vi "Build Channel Group.vi"(8 "error in":errorcluster, 9 "Selected Group":T1, 11 "Config Grandmaster":T3) -> (0 "error out":errorcluster={"status"=TRUE, "code"=-200220, "source"="Property Node DAQmx Device (arg 2) in ge_BuildGroup.vi <append>\n<B>Device Specified: </B>empty string"}, 1 "Selected Group":T1, 3 "Config Grandmaster":T3, 4 "Canceled?":bool)   [LabVIEW 2018, in "Configuration Grandmaster.lvlib" / "Cfg Grandmaster.lvclass"]
uses:
  Cfg Grandmaster.lvclass
  Custom Ctrls/ge_MeasType.ctl
  Custom Ctrls/Master Cfg/ge_Cfg wChassis.ctl
  Class Chassis Cfg/ChassisCfg.lvclass
  Class Chassis BOM/Chassis BOM.lvclass
  Data Acquisition/Class Chassis Tasks/Chassis Tasks.lvclass
  Common/Controls/Selected Group.ctl
  Common/Controls/TE_Designator.ctl
  Class Chassis BOM/Chassis BOM.lvclass/Chassis BOM.ctl
  <vilib>/Utility/miscctls.llb/LVRowAndColumnTypeDef.ctl
  <vilib>/Utility/miscctls.llb/LVRowAndColumnUnsignedTypeDef.ctl
  Class Chassis BOM/Read Mod Infos.vi
  Class Chassis BOM/Read Chassis Alias.vi
  Class Chan Group/Read GrpName.vi
  Class Chan Group/Read MeasType.vi
  <resource>/objmgr/daqmx.rc
  Measurements/Class Channel/Channel.lvclass
  Class Chan Group/ChanGrp.lvclass
panel:
  in  "Timing Engine":T2
  in  "MeasType":T4=enum."Dynamic"
  in  "Cancel":bool
  in  "Apply":bool
  in  "Group Name":string
  in  "Multicolumn Listbox":i32[](listbox)
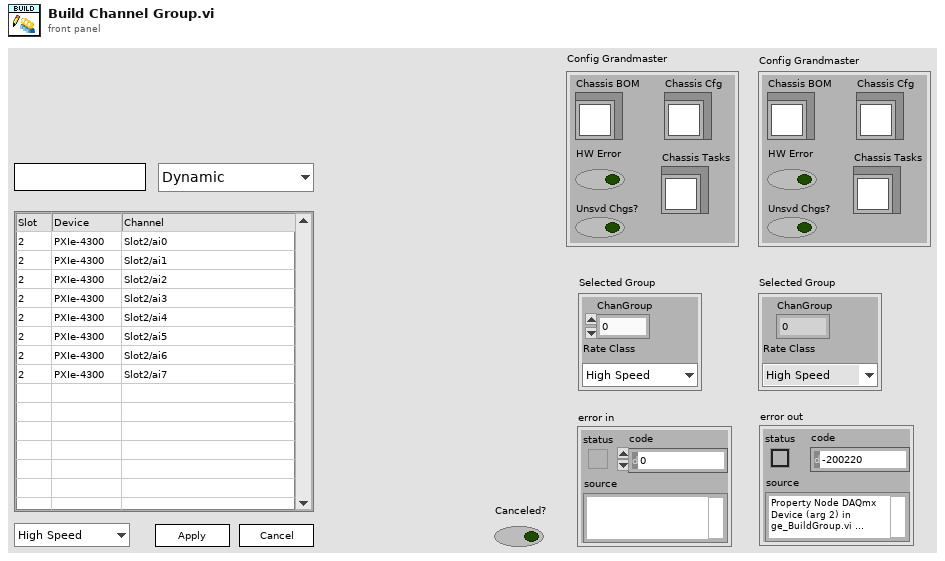
[diagram p1: front panel]
types:
  T1 = typedef "Selected Group.ctl" = cluster{"ChanGroup":i32, "Rate Class":T2}
  T2 = typedef "TE_Designator.ctl" = enum16{"High Speed", "Low Speed"}
  T3 = typedef "ge_Cfg wChassis.ctl" = cluster{"Chassis BOM":refnum<class "Chassis BOM.lvclass">, "Chassis Cfg":refnum<class "ChassisCfg.lvclass">, "Chassis Tasks":refnum<class "Chassis Tasks.lvclass">, "HW Error":bool, "Unsvd Chgs?":bool}
  T4 = typedef "ge_MeasType.ctl" = enum16{"Voltage", "Frequency", "Tachometer", "Dynamic", "Thermocouple", "RTD", "Strain", "Current", "Resistance"}
  T5 = typedef "Configuration Grandmaster.lvlib/Chassis BOM.lvclass/DAQmx Mod Info.ctl" = cluster{"Slot Number":i32, "DAQmx Alias":string}
  T6 = typedef "LVRowAndColumnUnsignedTypeDef.ctl" = cluster{"Row":u32, "Column":u32}
  T7 = typedef "LVRowAndColumnTypeDef.ctl" = cluster{"Row":i32, "Column":i32}
  T8 = enum8{"Enabled", "Disabled", "Disabled and Grayed Out"}
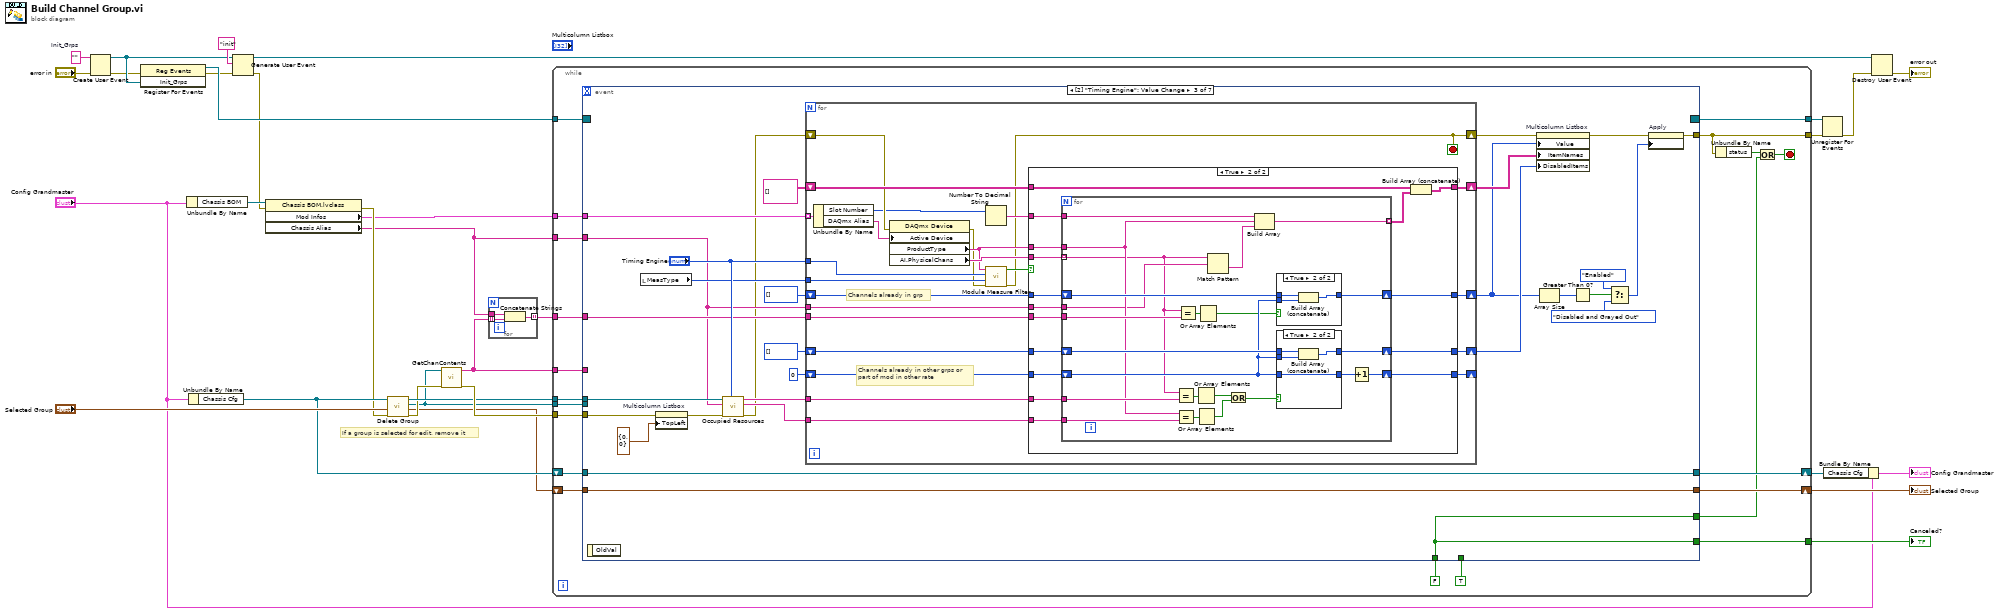
[diagram p0: block diagram]
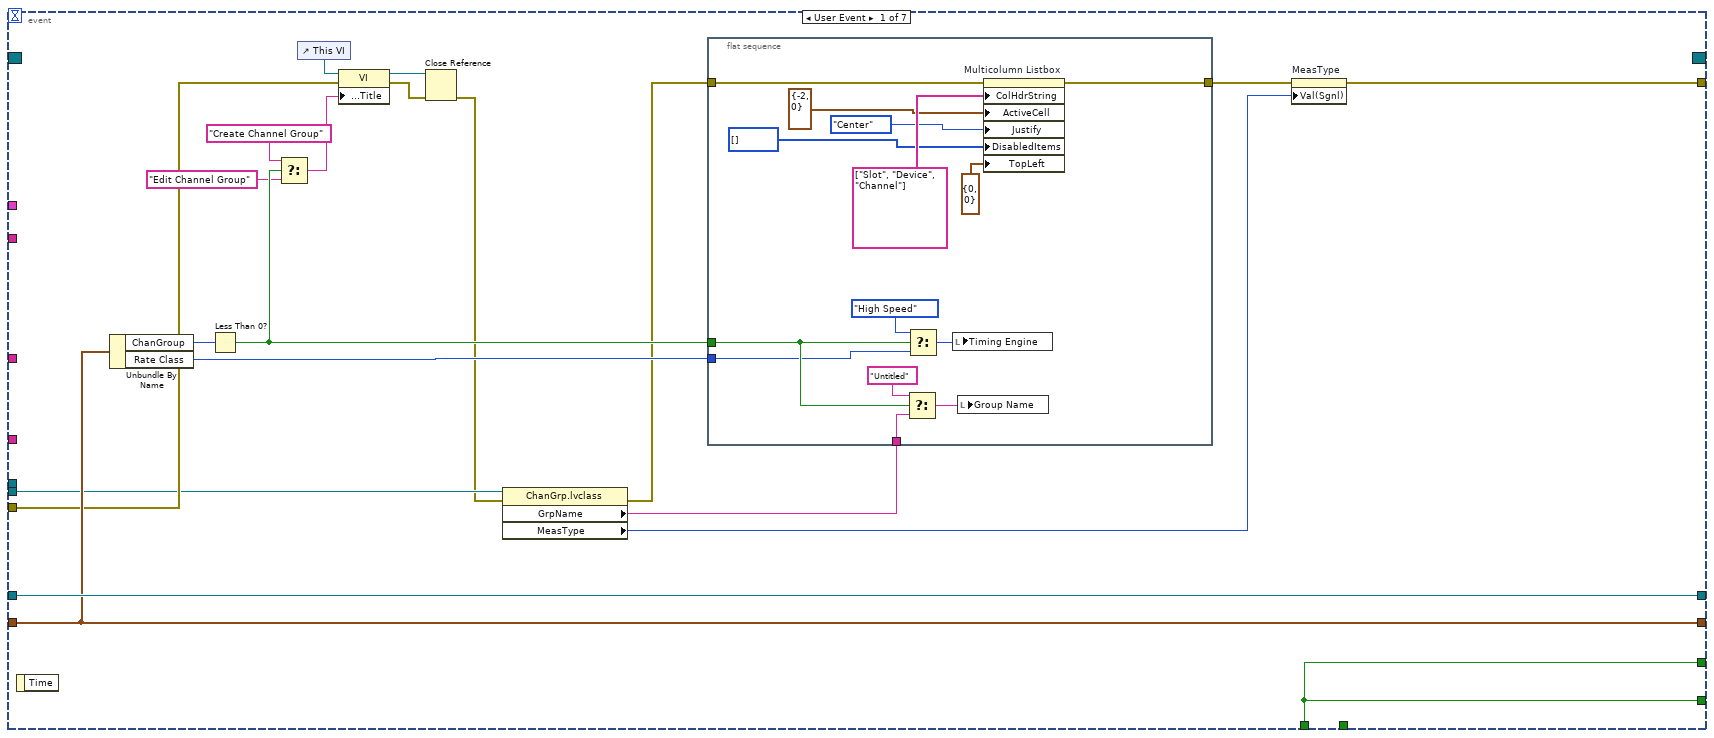
[diagram p2: hidden frame]
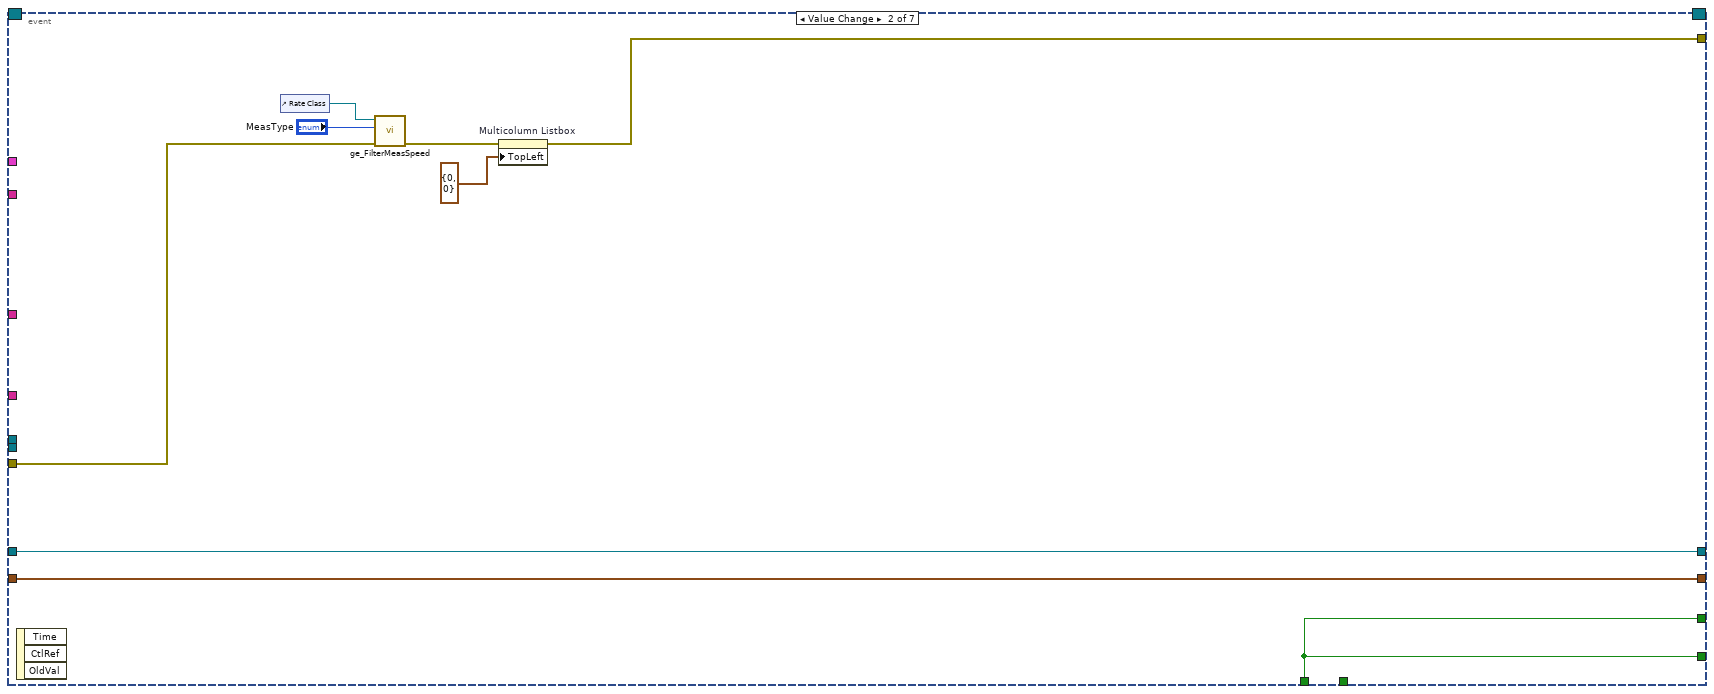
[diagram p3: hidden frame]
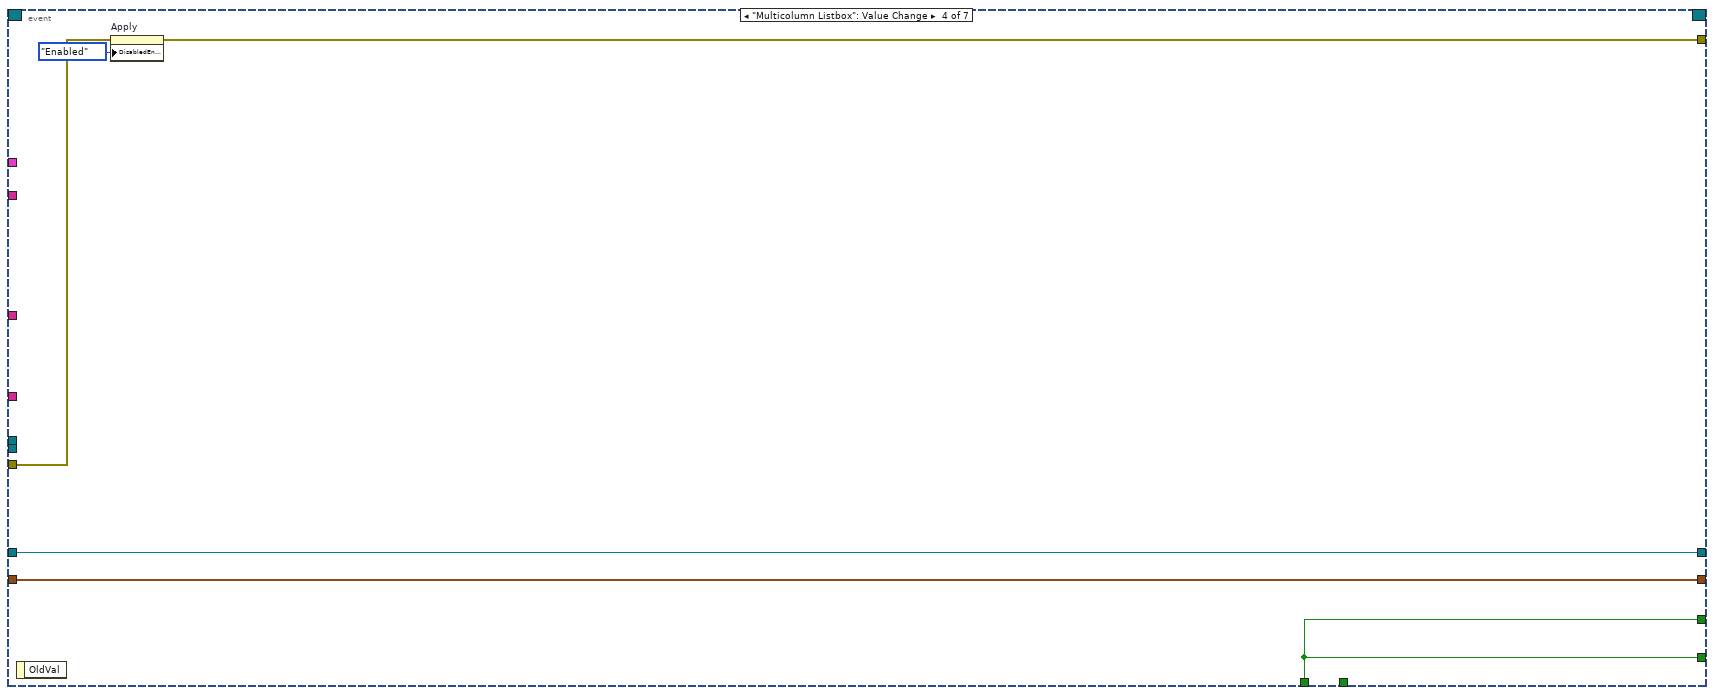
[diagram p7: hidden frame]
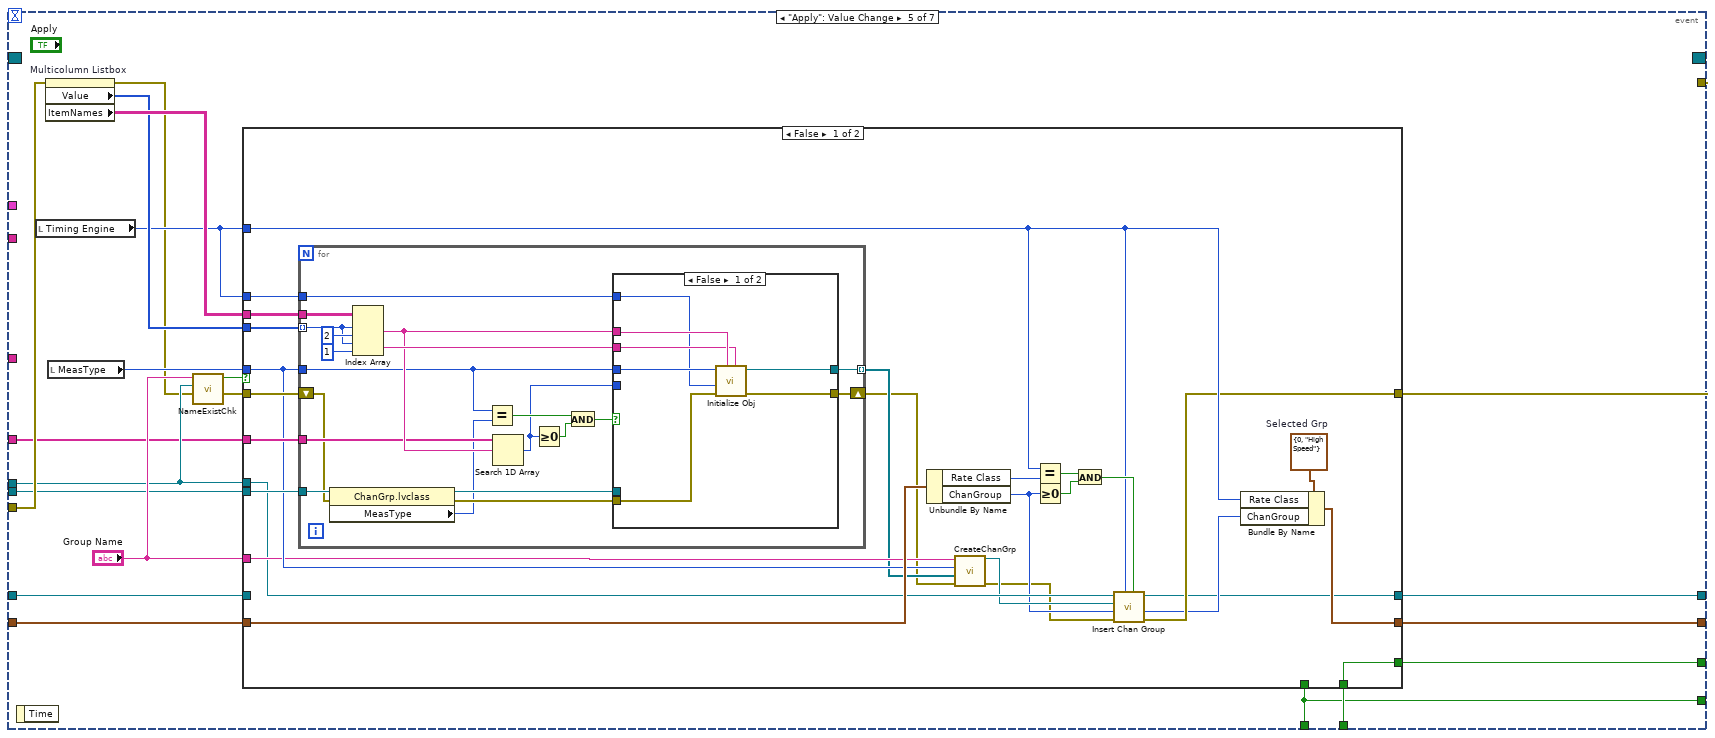
[diagram p8: hidden frame]
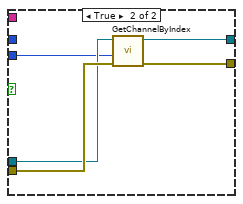
[diagram p9: hidden frame]
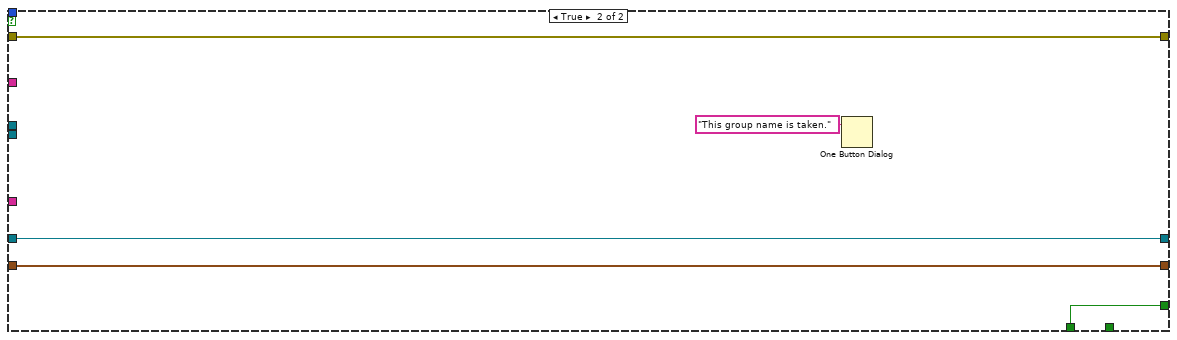
[diagram p10: hidden frame]
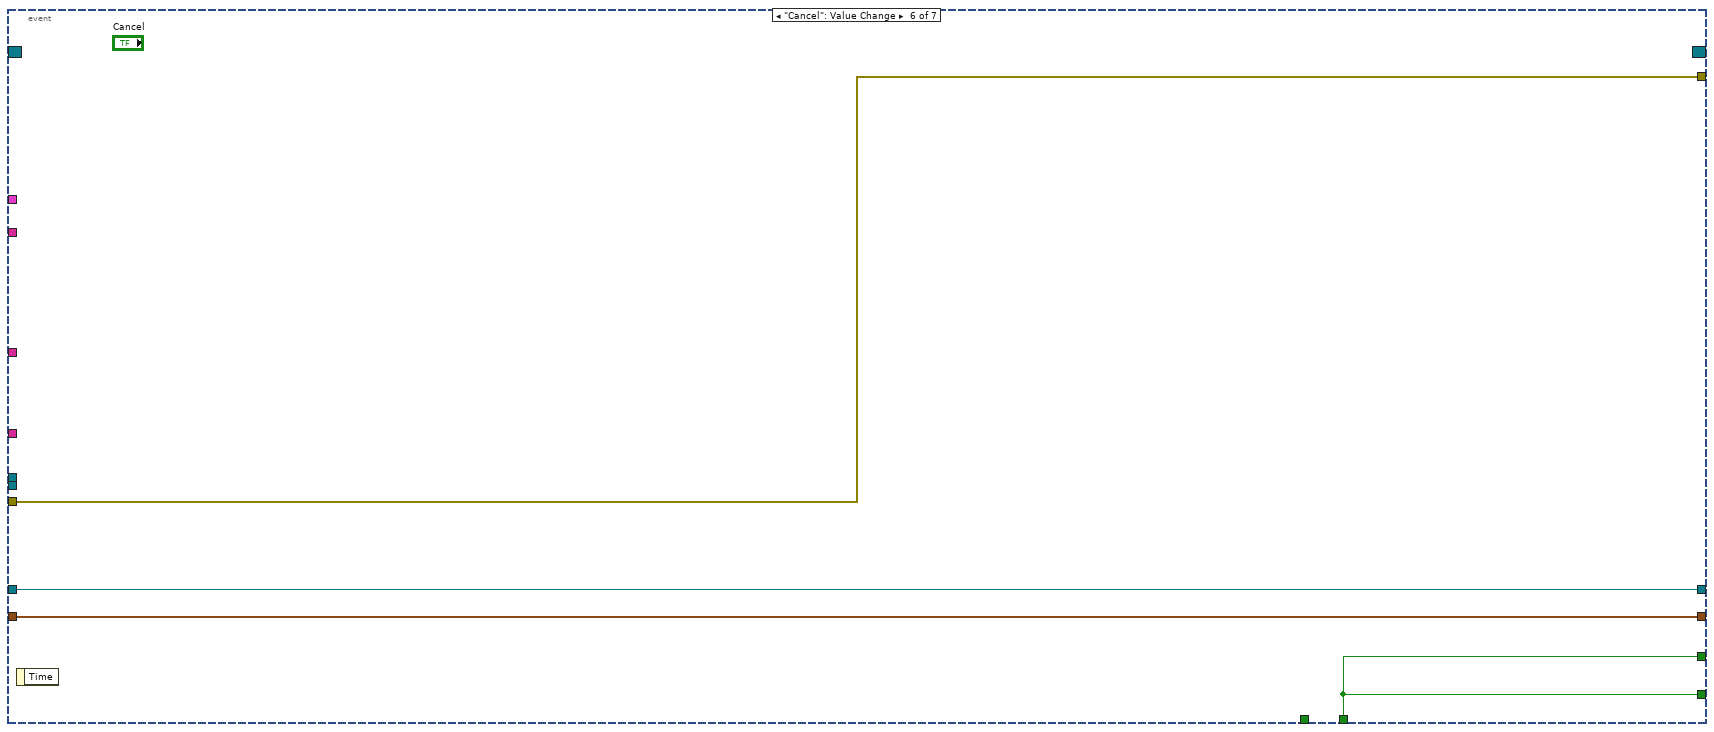
[diagram p11: hidden frame]
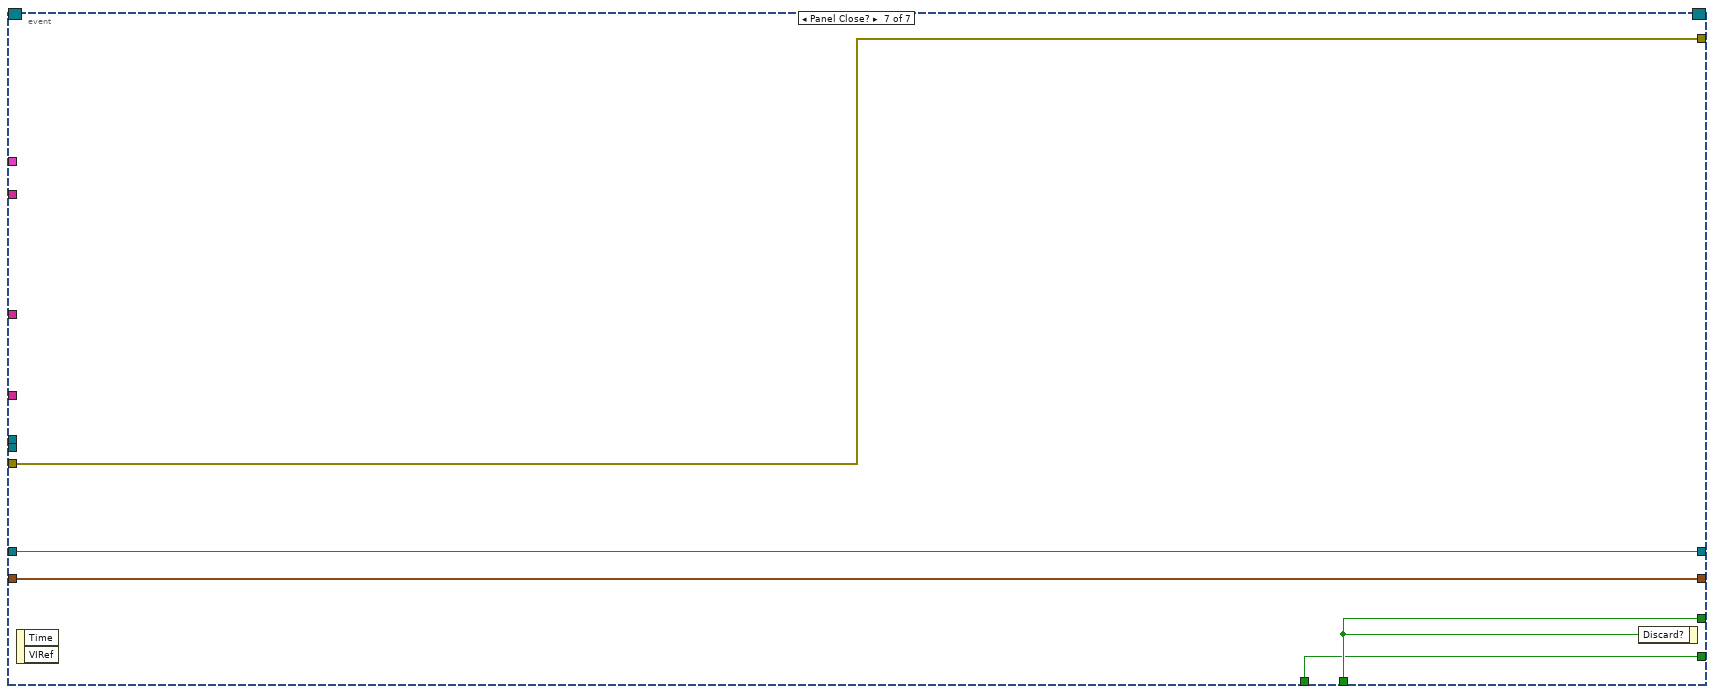
[diagram p12: hidden frame]
diagram:
  w19 = ""  # Init_Grps
  # "If a group is selected for edit, remove it"
  n1 = Create User Event(user event datatype=w19, error in="error in") -> (user event=w17:refnum<user-event>, error out=w16:errorcluster)
  n2 = register-events(error in=w16, w17) -> (reference out=w30:refnum<event-registration>, error out=w18:errorcluster)  [unwired: 1 in]
  n3 = Unbundle By Name("Config Grandmaster") -> ("Chassis BOM"=w6:refnum<class "Chassis BOM.lvclass">)
  n4 = Unbundle By Name("Config Grandmaster") -> ("Chassis Cfg"=w14:refnum<class "ChassisCfg.lvclass">)
  n5 = Generate User Event(user event=w17, event data cluster="init" ("event data"), error in=w18) -> (user event out=w27:refnum<user-event>, error out=w4:errorcluster)  [unwired: 1 in]
  n6 = property class="Chassis BOM.lvclass"(reference=w6, error in=w4) -> (error out=w5:errorcluster, "Mod Infos"=w3:T5[], "Chassis Alias"=w2:string)  [unwired: 1 out]
  n7 = call "Delete Group.vi"("error in"=w5, "Selected Group"="Selected Group", "Chassis Cfg"=w14) -> ("error out"=w10:errorcluster, "Selected Group"=w7:T1, "Deleted Grp"=w9:refnum<class "ChanGrp.lvclass">, "Chassis Cfg"=w22:refnum<class "ChassisCfg.lvclass">)  [unwired: 5 in]
  n8 = call "GetChanContents.vi"("error in"=w10, "ChanGrp.lvclass"=w9) -> ("error out"=w31:errorcluster, "All GrpChan Names"=w8:string[])  [unwired: 3 in, 5 out]
  n9 = for {
    tunnel: [w34] -> w11 mode=indexing
    tunnel: w2 -> [w33]
    tunnel: w8 -> [w32] mode=indexing
    n10 = Concatenate Strings(w33, w32) -> (w34:string)
  }
  n11 = while {
    tunnel: w30 -> [w54]
    tunnel: [w53] -> w28
    tunnel: w31 -> [w52]
    tunnel: [w40] -> w24
    shift-right: [w51] -> w13
    shift-left: w14 -> [w50]
    tunnel: w22 -> [w49]
    shift-right: [w47] -> w23
    shift-left: w7 -> [w48]
    tunnel: w9 -> [w46]
    tunnel: [w43] -> w15
    tunnel: w2 -> [w42]
    tunnel: w3 -> [w41]
    tunnel: w8 -> [w36]
    tunnel: w11 -> [w35]
    stop <- w38 stop-if-true
    n12 = event shown="[2] \"Timing Engine\": Value Change" {
      selector: w54 -> [_ _ _ _ _ _ _]
      dyn-events: [_ _ _ _ _ _ _] -> w53
      timeout: _ -> [_ _ _ _ _ _ _]
      tunnel: [w68 w94 w106 w205 w220 w294 w302] -> w37
      tunnel: w52 -> [w65 w97 w102 w209 w230 w297 w301]
      tunnel: [w69 w90 w114 w208 w213 w297 w301] -> w40
      tunnel: w50 -> [w73 w96 w120 w207 w224 w296 w300]
      tunnel: [w73 w96 w120 w207 w227 w296 w300] -> w51
      tunnel: w49 -> [_ _ w109 _ w218 _ _]
      tunnel: w48 -> [w71 w95 w119 w206 w225 w295 w299]
      tunnel: [w71 w95 w119 w206 w228 w295 w299] -> w47
      tunnel: w46 -> [w59 _ _ _ w216 _ _]
      tunnel: FALSE -> [w68 w94 w106 w205 w217 _ w298]
      tunnel: TRUE -> [_ _ _ _ w221 w294 w302]
      tunnel: [w68 w94 w106 w205 w217 w294 w298] -> w43
      tunnel: w42 -> [_ _ w100 _ _ _ _]
      tunnel: w41 -> [_ _ w105 _ _ _ _]
      tunnel: w36 -> [_ _ _ _ w215 _ _]
      tunnel: w35 -> [_ _ w101 _ _ _ _]
      event User Event {
        n13 = event-data() -> ()  [unwired: 1 in, 1 out]
        n14 = Unbundle By Name(w71) -> ("ChanGroup"=w72:i32, "Rate Class"=w70:T2)
        n15 = Less Than 0?(x=w72) -> (x < 0?=w61:bool)
        n16 = Select(t="Create Channel Group", s=w61, f="Edit Channel Group") -> (s? t:f=w62:string)
        n17 = control-ref of="This VI"() -> (w64:refnum<vi>)
        n18 = property class="VI"(reference=w64, error in=w65, "Front Panel.Title"=w62) -> (reference out=w67:refnum<vi>, error out=w66:errorcluster)
        n19 = Close Reference(reference=w67, error in (no error)=w66) -> (error out=w56:errorcluster)
        n20 = property class="ChanGrp.lvclass"(reference=w59, error in=w56) -> (error out=w55:errorcluster, "GrpName"=w58:string, "MeasType"=w57:T4)  [unwired: 1 out]
        n21 = flat-sequence {
          tunnel: w55 -> [w84]
          tunnel: [w83] -> w74
          tunnel: w61 -> [w77]
          tunnel: w70 -> [w76]
          tunnel: w58 -> [w75]
          frame #0 {
            n22 = Select(t="Untitled", s=w77, f=w75) -> (s? t:f=w80:string)
            n23 = Select(t=TE_Designator."High Speed", s=w77, f=w76) -> (s? t:f=w79:T2)
            n24 = local write "Timing Engine"(w79) -> ()
            n25 = local write "Group Name"(w80) -> ()
            n26 = property on="Multicolumn Listbox" class="MCListbox (strict)"(error in=w84, "ColHdrString"=string[] ["Slot", "Device", "Channel"] ("Column Header Strings[]"), "ActiveCell"=T7 {"Row"=-2, "Column"=0} ("Active Cell:Active Cell"), "Justify"=enum16{"Left", "Center", "Right"}."Center" ("Active Cell:Cell Justification"), "DisabledItems"=i32[] [] ("Disabled Items"), "TopLeft"=T6 {"Row"=0, "Column"=0} ("Top Left Visible Cell")) -> (error out=w83:errorcluster)  [unwired: 1 in, 1 out]
          }
        }
        n27 = property on="MeasType" class="Enum (strict)"(error in=w74, "Val(Sgnl)"=w57) -> (error out=w69:errorcluster)  [unwired: 1 in, 1 out]
      }
      event Value Change {
        n28 = event-data() -> ()  [unwired: 1 in, 3 out]
        n29 = control-ref of="Rate Class"() -> (w93:refnum<vi>)
        n30 = call "ge_FilterMeasSpeed.vi"("error in"=w97, "MeasType"="MeasType", "Rate Class"=w93) -> ("error out"=w91:errorcluster)  [unwired: 8 in]
        n31 = property on="Multicolumn Listbox" class="MCListbox (strict)"(error in=w91, "TopLeft"=T6 {"Row"=0, "Column"=0} ("Top Left Visible Cell")) -> (error out=w90:errorcluster)  [unwired: 1 in, 1 out]
      }
      event Value Change {
        n32 = event-data() -> ()  [unwired: 1 in, 1 out]
        n33 = local read "MeasType"() -> (w104:T4)
        n34 = property on="Multicolumn Listbox" class="MCListbox (strict)"(error in=w102, "TopLeft"=T6 {"Row"=0, "Column"=0} ("Top Left Visible Cell")) -> (error out=w99:errorcluster)  [unwired: 1 in, 1 out]
        n35 = call "Occupied Resources.vi"("Rate Class"="Timing Engine", "error in"=w99, "Chassis Name"=w100, "Chassis Cfg"=w109) -> ("error out"=w98:errorcluster, "Taken Dual Rate Mods"=w108:string[], "All Chassis/Chan Names"=w118:string[])  [unwired: 5 in]
        n36 = for {
          shift-right: [w147] -> w123
          shift-left: string[][] [] -> [w148]
          tunnel: w104 -> [w146]
          shift-right: [w131] -> w127
          shift-left: w98 -> [w145]
          shift-right: [w142] -> w122
          shift-left: i32[] [] ("Disabled Items") -> [w143]
          shift-right: [w140] -> _
          shift-left: 0 -> [w141]
          shift-right: [w138] -> w117
          shift-left: i32[] [] ("Disabled Items") -> [w139]
          tunnel: w118 -> [w137]
          tunnel: "Timing Engine" -> [w136]
          tunnel: w108 -> [w135]
          tunnel: w101 -> [w134]
          tunnel: w100 -> [w133]
          tunnel: w105 -> [w130] mode=indexing
          stop <- w131 stop-if-true
          # "Channels already in other grps or\npart of mod in other rate"
          # "Channels already in grp"
          n37 = Unbundle By Name(w130) -> ("Slot Number"=w128:i32, "DAQmx Alias"=w129:string)
          n38 = property class="DAQmx Device"(error in=w145, "Active Device"=w129) -> (error out=w132:errorcluster, "ProductType"=w149:string, "AI.PhysicalChans"=w151:tag[])  [unwired: 1 in, 1 out]
          n39 = Number To Decimal String(number=w128) -> (decimal integer string=w150:string)  [unwired: 1 in]
          n40 = call "Module Measure Filter.vi"("error in"=w132, "MeasType"=w146, "Rate Class"=w136, "Module Name"=w149) -> ("error out"=w131:errorcluster, "Mod Pass"=w144:bool)  [unwired: 6 in]
          n41 = case shown="True" w144 {
            tunnel: w151 -> [_ w171]
            tunnel: w150 -> [_ w170]
            tunnel: w149 -> [_ w169]
            tunnel: w148 -> [w155 w168]
            tunnel: [w155 w166] -> w147
            tunnel: w137 -> [_ w165]
            tunnel: w143 -> [w154 w164]
            tunnel: [w154 w163] -> w142
            tunnel: w141 -> [w153 w162]
            tunnel: [w153 w161] -> w140
            tunnel: w139 -> [w152 w160]
            tunnel: [w152 w159] -> w138
            tunnel: w134 -> [_ w158]
            tunnel: w135 -> [_ w157]
            tunnel: w133 -> [_ w156]
            frame False {
            }
            frame True {
              n42 = for {
                tunnel: w171 -> [w173] mode=indexing
                tunnel: w169 -> [w180]
                tunnel: w170 -> [w194]
                tunnel: [w193] -> w167 mode=indexing
                tunnel: w165 -> [w192]
                shift-right: [w190] -> w163
                shift-left: w164 -> [w191]
                shift-right: [w187] -> w161
                shift-left: w162 -> [w186]
                shift-right: [w184] -> w159
                shift-left: w160 -> [w185]
                tunnel: w158 -> [w181]
                tunnel: w157 -> [w179]
                tunnel: w156 -> [w174]
                n43 = Equal?(x=w173, y=w192) -> (x = y?=w189:bool[])
                n44 = Equal?(x=w180, y=w179) -> (x = y?=w178:bool[])
                n45 = Equal?(x=w173, y=w181) -> (x = y?=w183:bool[])
                n46 = Or Array Elements(Boolean array=w189) -> (logical OR=w177:bool)
                n47 = Or Array Elements(Boolean array=w178) -> (logical OR=w176:bool)
                n48 = Or Array Elements(Boolean array=w183) -> (logical OR=w182:bool)
                n49 = Match Pattern(string=w173, regular expression=w174) -> (after substring=w172:string)  [unwired: 1 in, 3 out]
                n50 = Or(x=w177, y=w176) -> (x .or. y?=w175:bool)
                n51 = Build Array(w194, w180, w172) -> (w193:string[])
                n52 = case shown="True" w182 {
                  tunnel: w185 -> [w195 w198]
                  tunnel: [w195 w197] -> w184
                  tunnel: w186 -> [_ w196]
                  frame False {
                  }
                  frame True {
                    n53 = Build Array (concatenate)(w198, w196) -> (w197:i32[])
                  }
                }
                n54 = case shown="True" w175 {
                  tunnel: w191 -> [w200 w204]
                  tunnel: w186 -> [w199 w202]
                  tunnel: [w200 w203] -> w190
                  tunnel: [w199 w202] -> w188
                  tunnel: w186 -> [_ w201]
                  frame False {
                  }
                  frame True {
                    n55 = Build Array (concatenate)(w204, w201) -> (w203:i32[])
                  }
                }
                n56 = Increment(x=w188) -> (x+1=w187:i32)
              }
              n57 = Build Array (concatenate)(w168, w167) -> (w166:string[][])
            }
          }
        }
        n58 = property on="Multicolumn Listbox" class="MCListbox (strict)"(error in=w127, "Value"=w117, "ItemNames"=w123, "DisabledItems"=w122) -> (error out=w115:errorcluster)  [unwired: 1 in, 1 out]
        n59 = Array Size(array=w117) -> (size(s)=w116:i32)
        n60 = Greater Than 0?(x=w116) -> (x > 0?=w107:bool)
        n61 = Select(t=T8."Enabled" ("Disabled"), s=w107, f=T8."Disabled and Grayed Out" ("Disabled")) -> (s? t:f=w111:T8)
        n62 = property on="Apply" class="Bool"(error in=w115, "DisabledEnum"=w111) -> (error out=w114:errorcluster)  [unwired: 1 in, 1 out]
      }
      event "Multicolumn Listbox": Value Change {
        n63 = event-data() -> ()  [unwired: 1 in, 1 out]
        n64 = property on="Apply" class="Bool"(error in=w209, "DisabledEnum"=T8."Enabled" ("Disabled")) -> (error out=w208:errorcluster)  [unwired: 1 in, 1 out]
      }
      event "Apply": Value Change {
        n65 = event-data() -> ()  [unwired: 1 in, 1 out]
        n66 = local read "Timing Engine"() -> (w214:T2)
        n67 = property on="Multicolumn Listbox" class="MCListbox (strict)"(error in=w230) -> (error out=w212:errorcluster, "Value"=w222:i32[], "ItemNames"=w229:string[][])  [unwired: 1 in, 1 out]
        n68 = local read "MeasType"() -> (w226:T4)
        n69 = call "NameExistChk.vi"("error in"=w212, "Chassis Cfg"=w218, "Group Name"="Group Name") -> ("error out"=w211:errorcluster, "Name Taken?"=w219:bool)  [unwired: 7 in]
        n70 = case shown="False" w219 {
          tunnel: w229 -> [w256 _]
          tunnel: w222 -> [w255 _]
          tunnel: [w253 w293] -> w228
          tunnel: [w231 w292] -> w227
          tunnel: w226 -> [w246 _]
          tunnel: w214 -> [w238 _]
          tunnel: "Group Name" -> [w245 _]
          tunnel: w225 -> [w252 w293]
          tunnel: w218 -> [w237 _]
          tunnel: w224 -> [_ w292]
          tunnel: [w251 w291] -> w220
          tunnel: w221 -> [w251 _]
          tunnel: w217 -> [_ w291]
          tunnel: w216 -> [w250 _]
          tunnel: w215 -> [w249 _]
          tunnel: w214 -> [w248 _]
          tunnel: w211 -> [w247 w289]
          tunnel: [w233 w289] -> w213
          frame False {
            w254 = T1 {"ChanGroup"=0, "Rate Class"=enum."High Speed"}  # Selected Grp
            n71 = for {
              tunnel: w256 -> [w276]
              tunnel: w255 -> [w274] mode=indexing
              tunnel: w246 -> [w259]
              tunnel: [w272] -> w244 mode=indexing
              tunnel: w250 -> [w263]
              tunnel: w249 -> [w266]
              tunnel: w248 -> [w264]
              shift-right: [w265] -> w243
              shift-left: w247 -> [w261]
              n72 = property class="ChanGrp.lvclass"(reference=w263, error in=w261) -> (reference out=w262:refnum<class "ChanGrp.lvclass">, error out=w260:errorcluster, "MeasType"=w258:T4)
              n73 = Index Array(array=w276, index (row) #1=w274, index (col) #1=2 ("disabled index (row)"), index (row) #2=w274, index (col) #2=1 ("disabled index (col)")) -> (element #1=w267:string, element #2=w271:string)
              n74 = Equal?(x=w259, y=w258) -> (x = y?=w270:bool)
              n75 = Search 1D Array(1D array=w266, element=w267) -> (index of element=w257:i32)  [unwired: 1 in]
              n76 = Greater Or Equal To 0?(x=w257) -> (x >= 0?=w269:bool)
              n77 = And(x=w270, y=w269) -> (x .and. y?=w268:bool)
              n78 = case shown="False" w268 {
                tunnel: [w278 w285] -> w272
                tunnel: w267 -> [w281 _]
                tunnel: w271 -> [w280 _]
                tunnel: w259 -> [w283 _]
                tunnel: w257 -> [_ w284]
                tunnel: w260 -> [w282 w288]
                tunnel: [w277 w287] -> w265
                tunnel: w264 -> [w279 _]
                tunnel: w262 -> [_ w286]
                frame False {
                  n79 = call "Initialize Obj.vi"("Device"=w280, "ChanName"=w281, "error in (no error)"=w282, "Timing Engine"=w279, "MeasType"=w283) -> ("error out"=w277:errorcluster, "Channel out"=w278:refnum<class "Channel.lvclass">)  [unwired: 5 in]
                }
                frame True {
                  n80 = call "GetChannelByIndex.vi"("error in (no error)"=w288, "index of element"=w284, "ChanGrp in"=w286) -> ("error out"=w287:errorcluster, "Channel"=w285:refnum<class "Channel.lvclass">)  [unwired: 7 in]
                }
              }
            }
            n81 = Unbundle By Name(w252) -> ("Rate Class"=w242:T2, "ChanGroup"=w235:i32)
            n82 = call "CreateChanGrp.vi"("error in (no error)"=w243, "GroupChans"=w244, "MeasType"=w246, "GroupName"=w245) -> ("error out"=w234:errorcluster, "ChanGrp out"=w236:refnum<class "ChanGrp.lvclass">)  [unwired: 6 in]
            n83 = Equal?(x=w238, y=w242) -> (x = y?=w241:bool)
            n84 = Greater Or Equal To 0?(x=w235) -> (x >= 0?=w240:bool)
            n85 = And(x=w241, y=w240) -> (x .and. y?=w239:bool)
            n86 = call "Insert Chan Group.vi"("Insert to Prev Place? (T)"=w239, "Timing Engine"=w238, "error in (no error)"=w234, "ChanGroupPos"=w235, "ChanGrp to Add"=w236, "ChassisCfg in"=w237) -> ("error out"=w233:errorcluster, "ChanGroupPos"=w232:i32, "ChassisCfg out"=w231:refnum<class "ChassisCfg.lvclass">)  [unwired: 3 in]
            n87 = Bundle By Name(cluster=w254, "Rate Class"=w238, "ChanGroup"=w232) -> (w253:T1)
          }
          frame True {
            n88 = One Button Dialog(message="This group name is taken.") -> ()  [unwired: 1 in, 1 out]
          }
        }
      }
      event "Cancel": Value Change {
        n89 = event-data() -> ()  [unwired: 1 in, 1 out]
      }
      event Panel Close? {
        n90 = event-data() -> ()  [unwired: 1 in, 2 out]
        n91 = event-data("Discard?"=w302) -> ()  [unwired: 1 in, 1 out]
      }
    }
    n92 = Unbundle By Name(w40) -> ("status"=w39:bool)
    n93 = Or(x=w39, y=w37) -> (x .or. y?=w38:bool)
  }
  "Selected Group" <- w23
  "Canceled?" <- w15
  n94 = Unregister For Events(event registration refnum=w28, error in=w24) -> (error out=w29:errorcluster)
  n95 = Bundle By Name(cluster="Config Grandmaster", "Chassis Cfg"=w13) -> (→"Config Grandmaster":T3)
  n96 = Destroy User Event(user event=w27, error in=w29) -> (error out=→"error out":errorcluster)
